vi "PMAC3000 SetUpDeviceOnUSB.vi"(0 "RD/WR Timeouts":i32=100, 1 "Software Number":string, 2 "VersionNumbers":string[](array[string]), 5 "Latency Timer":u8=8, 7 "Data Set-Up":T1={"Baud Rate"=1250000, "DataBits"=0, "StopBits"=0, "Parity"=0} {"Parity" items=["PARITY_NONE", "PARITY_ODD", "PARITY_EVEN", "PARITY_MARK", "PARITY_SPACE"]; "StopBits" items=["STOP_BITS_1", "STOP_BITS_1_5", "STOP_BITS_2"]; "DataBits" items=["BITS_5"=5, "BITS_6"=6, "BITS_7"=7, "BITS_8"=8]}, 9 "Flow Control Input":cluster{"FlowControl":u16, "Xon":u8, "Xoff":u8} {"FlowControl" items=["FLOW_NONE"=0, "FLOW_RTS_CTS"=256, "FLOW_DTR_DSR"=512, "FLOW_XON_OFF"=1024]}, 11 "Show Not Found Message":bool=TRUE, 12 "error in (no error)":errorcluster) -> (4 "USB Device Found":bool, 6 "USB Handle":i32, 8 "error out":errorcluster, 10 "NumberOfUsbDevices":i32, 14 "SoftwareVersionFound":string, 15 "Error":i32)   [LabVIEW 2018]
uses:
  ftd2xx.dll
panel:
  in  "FlowControl":u16(ring) items=["FLOW_NONE"=0, "FLOW_RTS_CTS"=256, "FLOW_DTR_DSR"=512, "FLOW_XON_OFF"=1024]
  in  "Parity":u8(ring) items=["PARITY_NONE", "PARITY_ODD", "PARITY_EVEN", "PARITY_MARK", "PARITY_SPACE"]
  in  "StopBits":u8(ring) items=["STOP_BITS_1", "STOP_BITS_1_5", "STOP_BITS_2"]
  in  "DataBits":u8(ring) items=["BITS_5"=5, "BITS_6"=6, "BITS_7"=7, "BITS_8"=8]
  out "Flags":i32
  out "Show Message":bool
  in  "Xoff":u8
  in  "Xon":u8
  in  "Baud Rate":i32=1250000
  out "Device Index":i32
  out "Number of Devices":i32
  # "Inputs"
  # "Misc"
  # "Outputs"
  # "e"
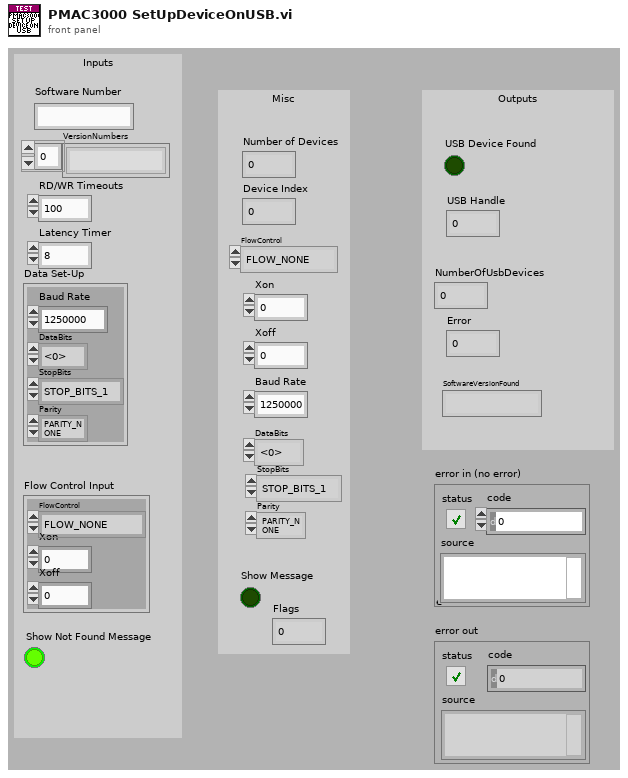
[diagram p1: front panel]
types:
  T1 = cluster{"Baud Rate":i32, "DataBits":u8, "StopBits":u8, "Parity":u8}
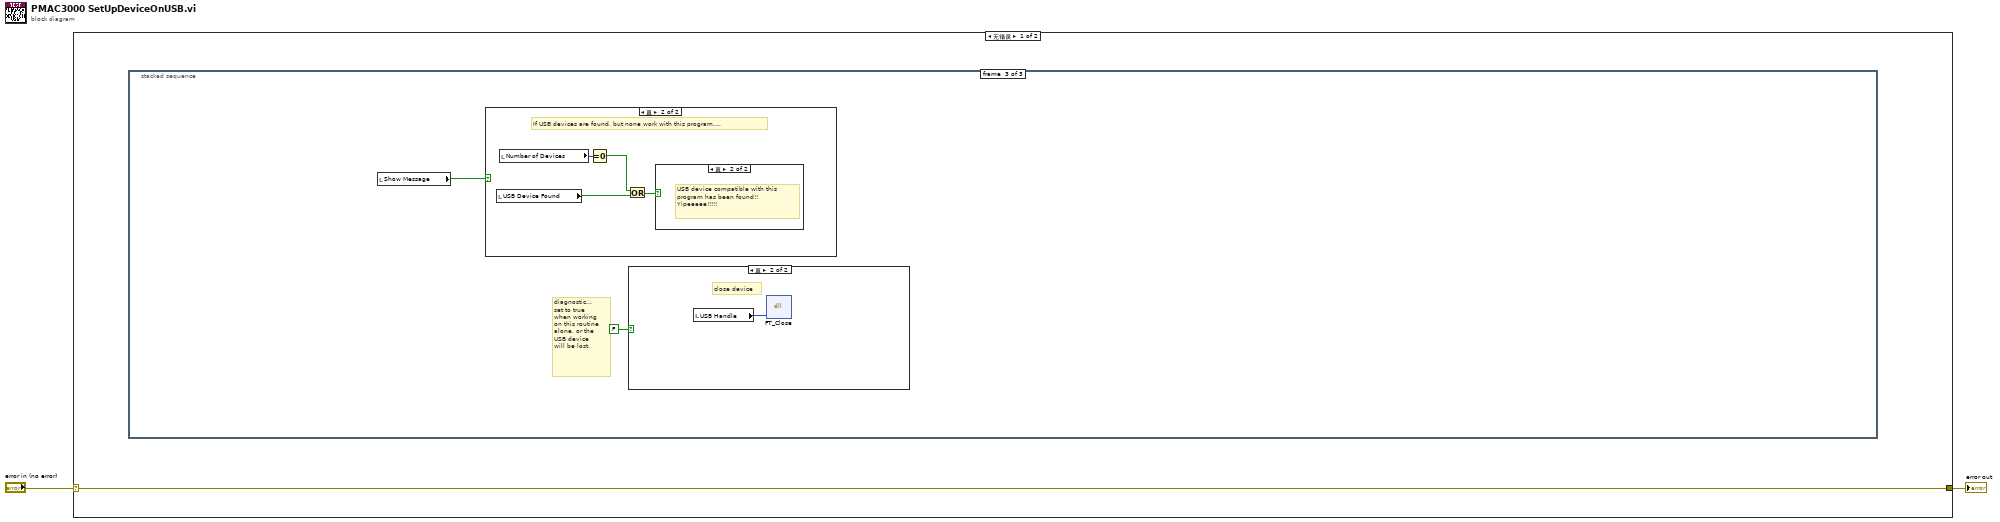
[diagram p0: block diagram]
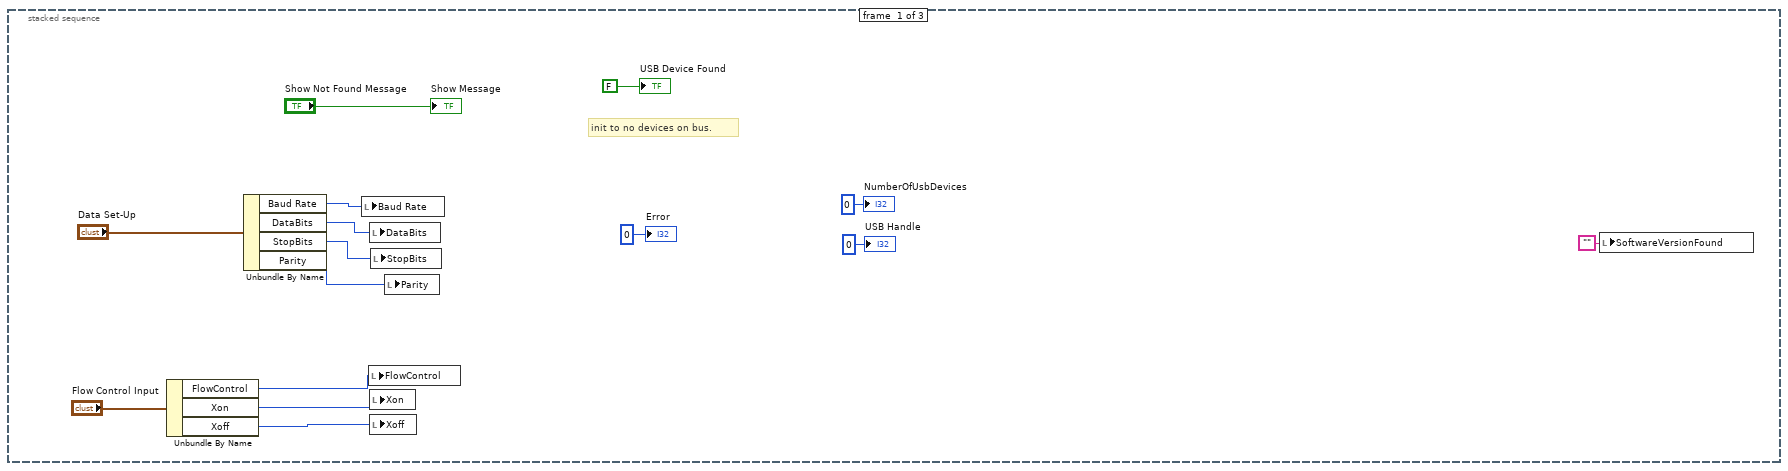
[diagram p2: hidden frame]
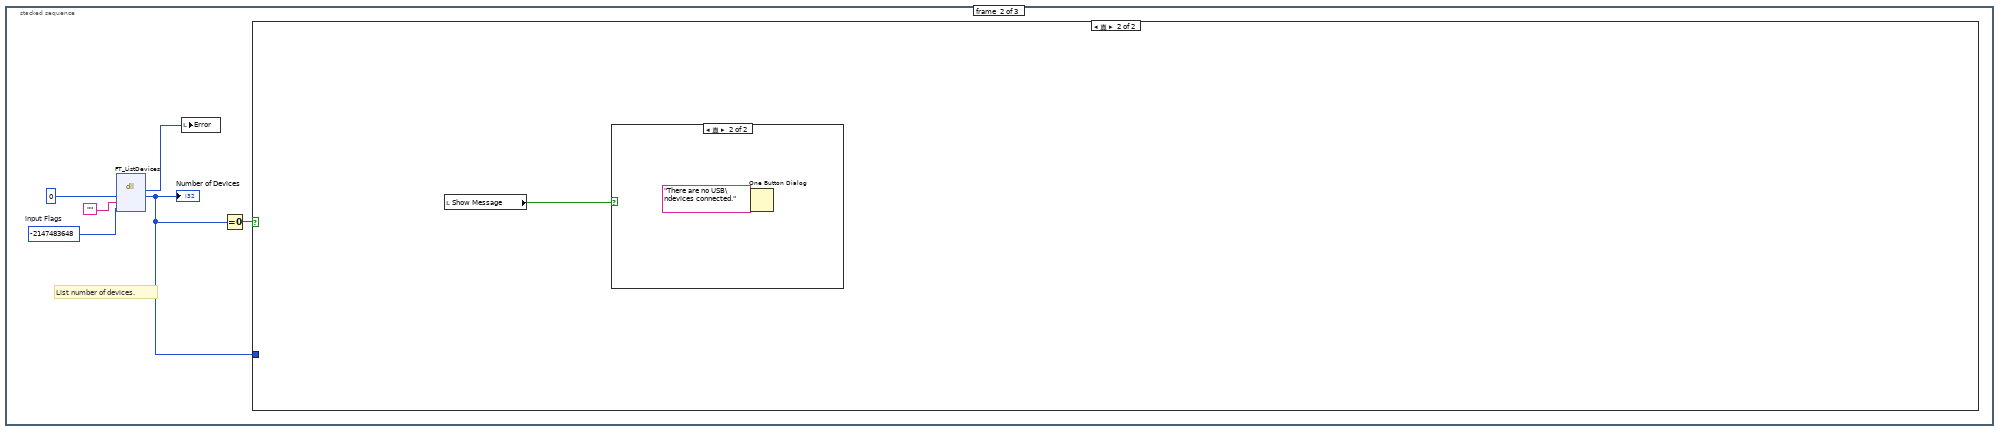
[diagram p3: hidden frame]
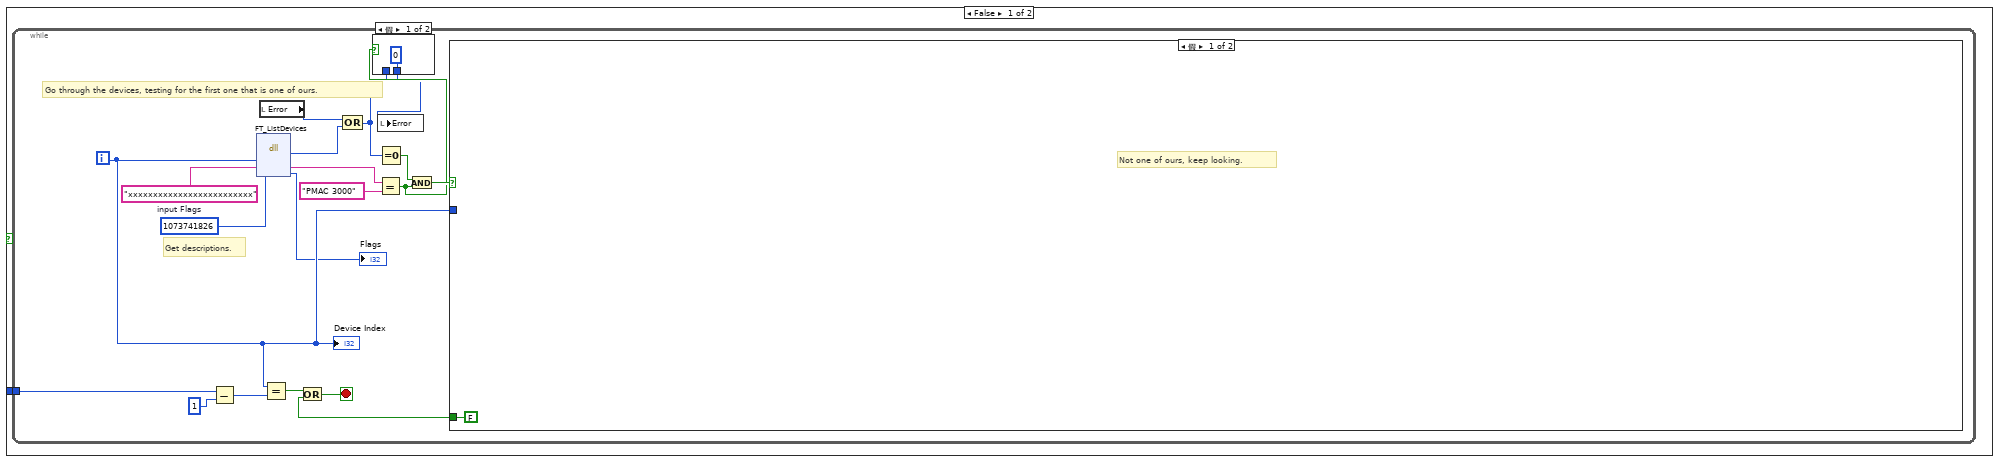
[diagram p4: hidden frame]
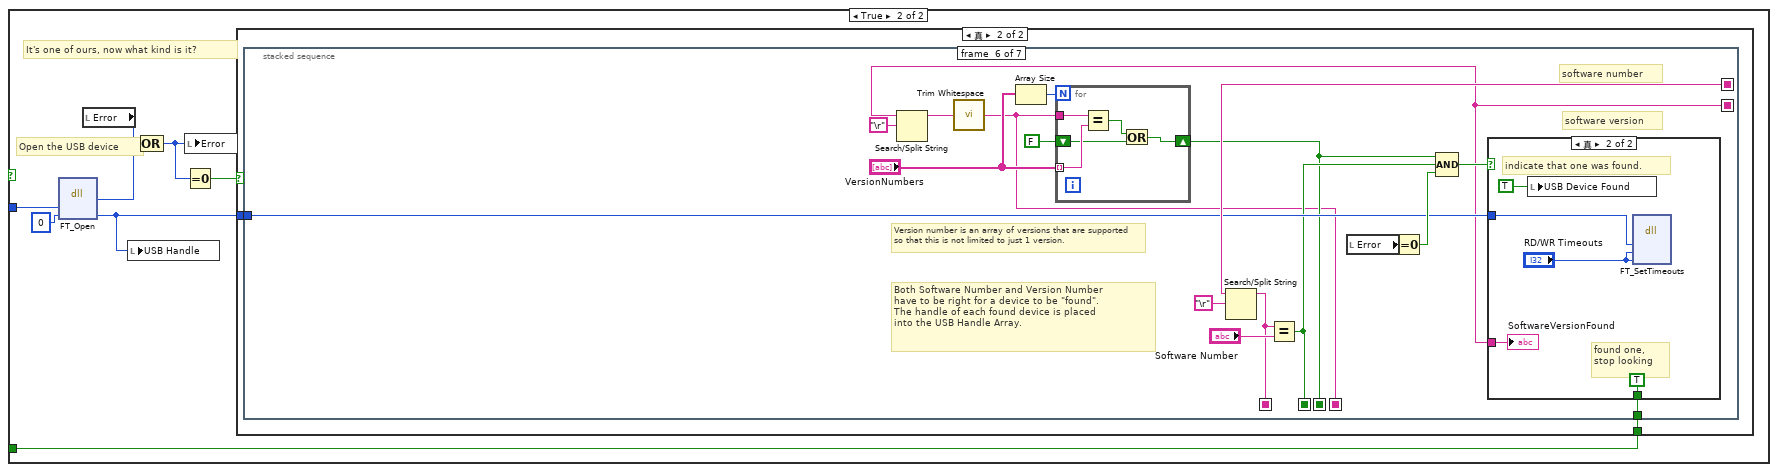
[diagram p6: hidden frame]
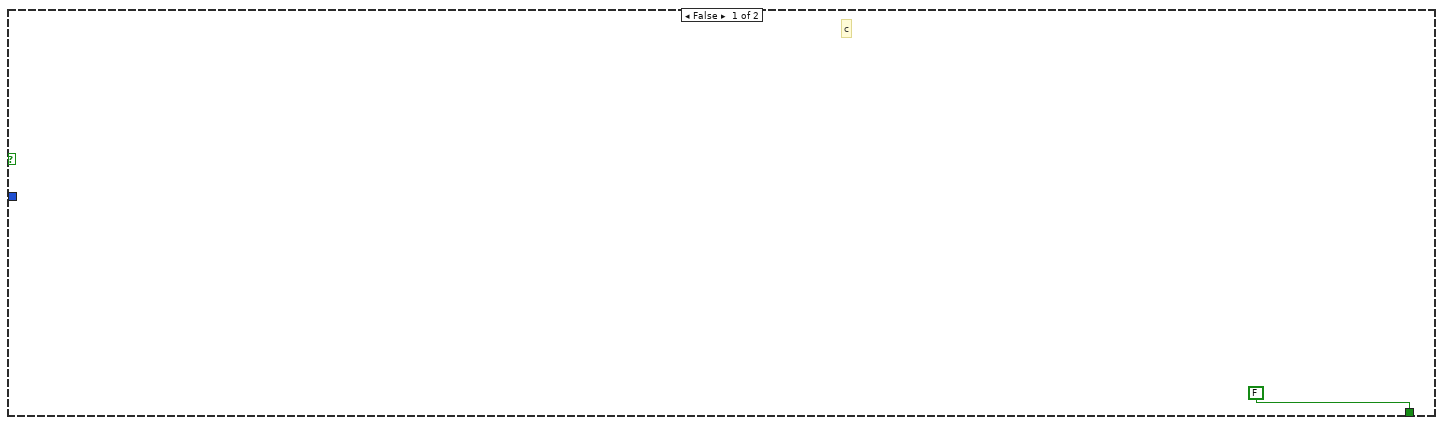
[diagram p7: hidden frame]
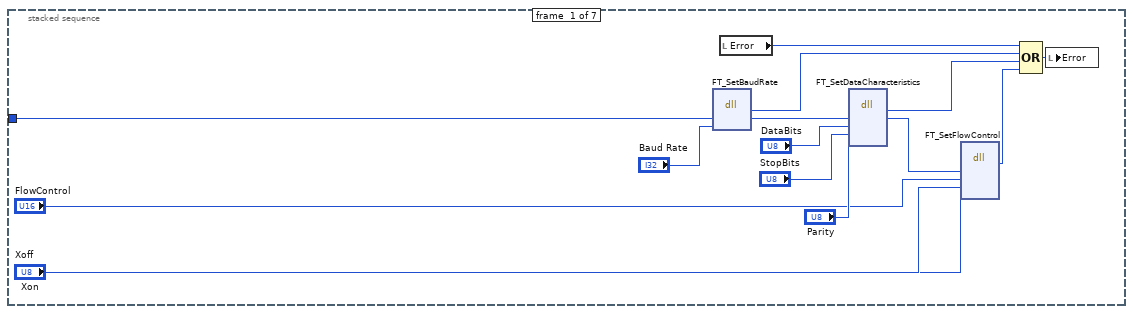
[diagram p8: hidden frame]
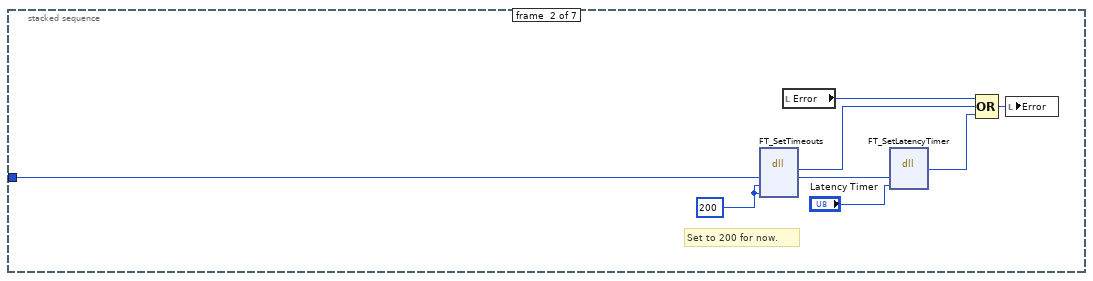
[diagram p9: hidden frame]
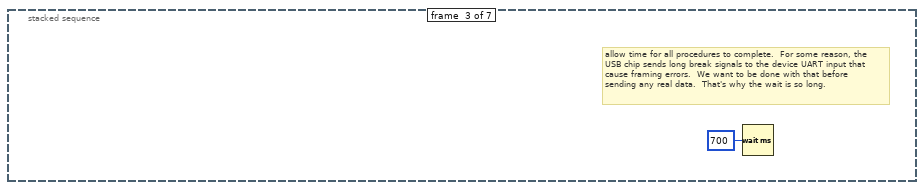
[diagram p10: hidden frame]
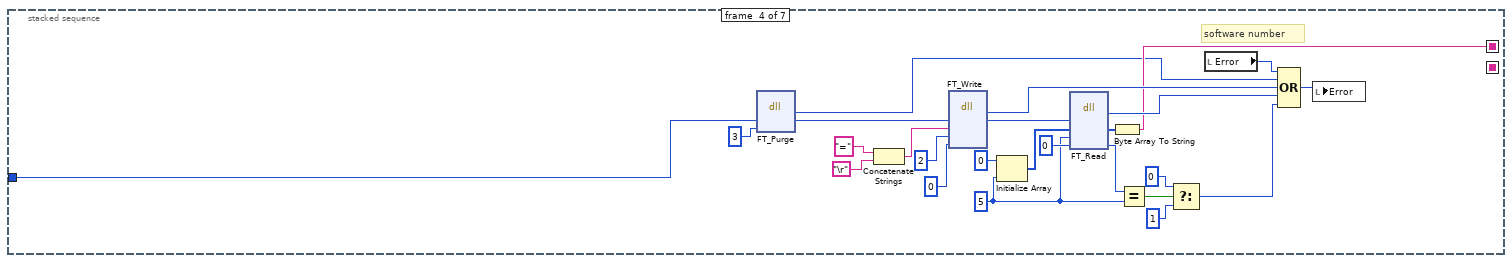
[diagram p11: hidden frame]
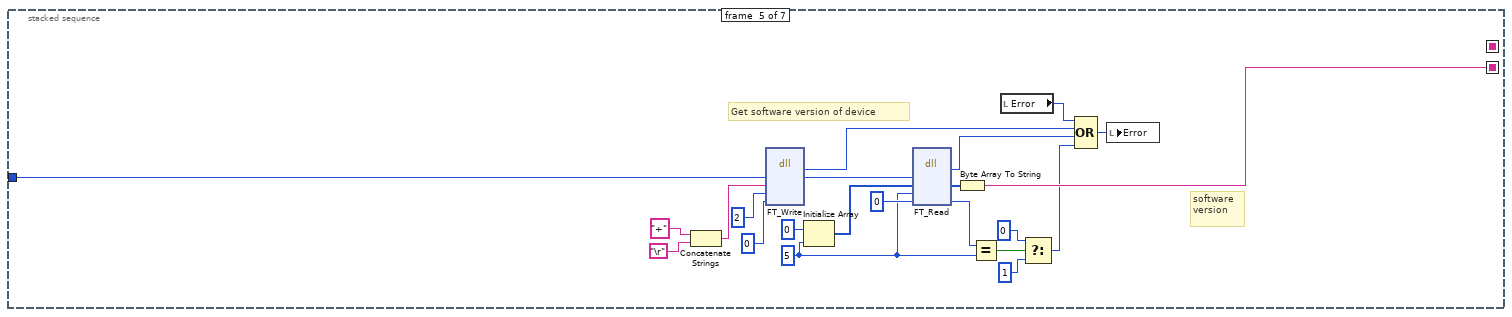
[diagram p12: hidden frame]
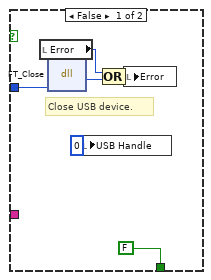
[diagram p13: hidden frame]
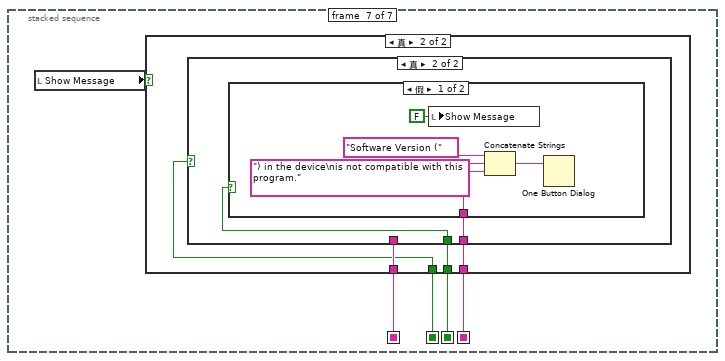
[diagram p14: hidden frame]
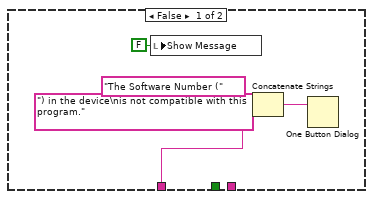
[diagram p16: hidden frame]
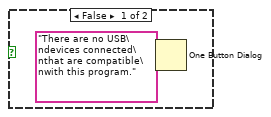
[diagram p20: hidden frame]
diagram:
  n1 = case shown="无错误" "error in (no error)" {
    selector: "error in (no error)" -> [w3 w195]
    tunnel: [w3 w195] -> w1
    frame No Error {
      n2 = stacked-sequence {
        frame #0 {
          # "init to no devices on bus."
          n3 = Unbundle By Name("Flow Control Input") -> ("FlowControl"=w6:u16, "Xon"=w5:u8, "Xoff"=w4:u8)
          n4 = Unbundle By Name("Data Set-Up") -> ("Baud Rate"=w11:i32, "DataBits"=w10:u8, "StopBits"=w9:u8, "Parity"=w8:u8)
          n5 = local write "Baud Rate"(w11) -> ()
          n6 = local write "FlowControl"(w6) -> ()
          n7 = local write "DataBits"(w10) -> ()
          n8 = local write "Xon"(w5) -> ()
          n9 = local write "Xoff"(w4) -> ()
          n10 = local write "StopBits"(w9) -> ()
          n11 = local write "Parity"(w8) -> ()
          n12 = local write "SoftwareVersionFound"("") -> ()
          "USB Device Found" <- FALSE ("USB Sensor Link Found")
          "Error" <- 0 ("Error")
          "Show Message" <- "Show Not Found Message"
          "NumberOfUsbDevices" <- 0 ("NumberOfUsbDevices")
          "USB Handle" <- 0 ("USB Handel")
        }
        frame #1 {
          w24 = -2147483648  # input Flags
          # "List number of devices."
          n13 = dll-call lib="C:/Labview Code/04.SubVI's/Others VI's/FTD2XX.dll" fn="FT_ListDevices"(0 ("input param"), "", "Flags"=w24) -> ("return type"=w19:i32, w21:i32)  [unwired: 5 in, 2 out]
          "Number of Devices" <- w21
          n14 = local write "Error"(w19) -> ()
          n15 = Equal To 0?(x=w21) -> (x = 0?=w23:bool)
          n16 = case shown="真" w23 {
            tunnel: w21 -> [w25 _]
            frame False {
              n17 = while {
                tunnel: w25 -> [w40]
                i -> [w38]
                stop <- w32 stop-if-true
                w43 = 1073741826  # input Flags
                # "Go through the devices, testing for the first one that is one of ours."
                # "Get descriptions."
                n18 = Subtract(x=w40, y=1) -> (x-y=w41:i32)
                n19 = dll-call lib="C:/Labview Code/04.SubVI's/Others VI's/FTD2XX.dll" fn="FT_ListDevices"(w38, "xxxxxxxxxxxxxxxxxxxxxxxxx" ("input param"), "Flags"=w43) -> ("return type"=w37:i32, w39:string, "Flags"=→"Flags":i32)  [unwired: 4 in, 2 out]
                n20 = local read "Error"() -> (w36:i32)
                n21 = Equal?(x=w38, y=w41) -> (x = y?=w33:bool)
                n22 = Compound Arithmetic op=OR(w36, w37) -> (w26:i32)
                n23 = Equal?(x=w39, y="PMAC 3000") -> (x = y?=w28:bool)
                n24 = case shown="假" w28 {
                  tunnel: [0 w46] -> w27
                  tunnel: w26 -> [_ w46]
                  frame False {
                  }
                  frame True {
                  }
                }
                n25 = local write "Error"(w27) -> ()
                n26 = Equal To 0?(x=w26) -> (x = 0?=w35:bool)
                n27 = And(x=w35, y=w28) -> (x .and. y?=w34:bool)
                n28 = case shown="假" w34 {
                  tunnel: w38 -> [_ w55]
                  tunnel: [FALSE w48] -> w31
                  frame False {
                    # "Not one of ours, keep looking."
                  }
                  frame True {
                    # "Open the USB device"
                    # "It's one of ours, now what kind is it?"
                    n29 = dll-call lib="C:/Labview Code/04.SubVI's/Others VI's/FTD2XX.dll" fn="FT_Open"(w55, "Handle"=0 ("input Handle")) -> ("return type"=w52:i32, "Handle"=w49:i32)  [unwired: 4 in, 2 out]
                    n30 = local read "Error"() -> (w53:i32)
                    n31 = local write "USB Handle"(w49) -> ()
                    n32 = Compound Arithmetic op=OR(w53, w52) -> (w50:i32)
                    n33 = local write "Error"(w50) -> ()
                    n34 = Equal To 0?(x=w50) -> (x = 0?=w51:bool)
                    n35 = case shown="真" w51 {
                      tunnel: w49 -> [_ w58]
                      tunnel: [FALSE w57] -> w48
                      frame False {
                        # "c"
                      }
                      frame True {
                        n36 = stacked-sequence {
                          seq-local: [_ _ _ w94 _ _ _] -> [_ _ _ _ _ w145 _]
                          seq-local: [_ _ _ _ w114 _ _] -> [_ _ _ _ _ w135 _]
                          seq-local: [_ _ _ _ _ w134 _] -> [_ _ _ _ _ _ w165]
                          seq-local: [_ _ _ _ _ w133 _] -> [_ _ _ _ _ _ w168]
                          seq-local: [_ _ _ _ _ w130 _] -> [_ _ _ _ _ _ w167]
                          seq-local: [_ _ _ _ _ w132 _] -> [_ _ _ _ _ _ w166]
                          tunnel: w58 -> [w63 w75 _ w93 w115 w140 _]
                          tunnel: [_ _ _ _ _ w139 _] -> w57
                          frame #0 {
                            n37 = dll-call lib="C:/Labview Code/04.SubVI's/Others VI's/FTD2XX.dll" fn="FT_SetBaudRate"("Handle"=w63, "BaudRate"="Baud Rate") -> ("return type"=w70:i32, "Handle"=w73:i32)  [unwired: 4 in, 2 out]
                            n38 = local read "Error"() -> (w69:i32)
                            n39 = dll-call lib="C:/Labview Code/04.SubVI's/Others VI's/FTD2XX.dll" fn="FT_SetDataCharacteristics"("Handle"=w73, "WordLength"="DataBits", "StopBits"="StopBits", "Parity"="Parity") -> ("return type"=w71:i32, "Handle"=w65:i32)  [unwired: 6 in, 2 out]
                            n40 = dll-call lib="C:/Labview Code/04.SubVI's/Others VI's/FTD2XX.dll" fn="FT_SetFlowControl"("Handle"=w65, "FlowControl"="FlowControl", "Xon"="Xon", "Xoff"="Xoff") -> ("return type"=w64:i32)  [unwired: 7 in, 2 out]
                            n41 = Compound Arithmetic op=OR(w69, w70, w71, w64) -> (w68:i32)
                            n42 = local write "Error"(w68) -> ()
                          }
                          frame #1 {
                            w74 = 200 ("RD/WR Timeouts")
                            # "Set to 200 for now."
                            n43 = dll-call lib="C:/Labview Code/04.SubVI's/Others VI's/FTD2XX.dll" fn="FT_SetTimeouts"("Handle"=w75, "ReadTimeout"=w74, "WriteTimeout"=w74) -> ("return type"=w78:i32, "Handle"=w81:i32)  [unwired: 5 in, 2 out]
                            n44 = local read "Error"() -> (w77:i32)
                            n45 = dll-call lib="C:/Labview Code/04.SubVI's/Others VI's/FTD2XX.dll" fn="FT_SetLatencyTimer"("Handle"=w81, "Timer"="Latency Timer") -> ("return type"=w79:i32)  [unwired: 5 in, 2 out]
                            n46 = Compound Arithmetic op=OR(w77, w78, w79) -> (w76:i32)
                            n47 = local write "Error"(w76) -> ()
                          }
                          frame #2 {
                            # "allow time for all procedures to complete.  For some reason, the\nUSB chip sends long break signals to the device UART input that\ncause framing errors.  We want to be done with that before\nsending any real data.  That's why the wait is so long."
                            n48 = Wait (ms)(milliseconds to wait=u32 700) -> ()  [unwired: 1 out]
                          }
                          frame #3 {
                            w87 = 5 ("dimension size")
                            # "software number"
                            n49 = dll-call lib="C:/Labview Code/04.SubVI's/Others VI's/FTD2XX.dll" fn="FT_Purge"("Handle"=w93, "Mask"=3) -> ("return type"=w90:i32, "Handle"=w92:i32)  [unwired: 4 in, 2 out]
                            n50 = Concatenate Strings("=" ("string"), "\r") -> (w106:string)
                            n51 = dll-call lib="C:/Labview Code/04.SubVI's/Others VI's/FTD2XX.dll" fn="FT_Write"("Handle"=w92, "Buffer"=w106, "BytesToWrite"=2, "BytesWritten"=0) -> ("return type"=w97:i32, "Handle"=w102:i32)  [unwired: 6 in, 2 out]
                            n52 = Initialize Array(u8 0 ("element"), w87) -> (w100:u8[])
                            n53 = dll-call lib="C:/Labview Code/04.SubVI's/Others VI's/FTD2XX.dll" fn="FT_Read"("Handle"=w102, "Buffer"=w100, "BytesToRead"=w87, "BytesReturned"=0) -> ("return type"=w96:i32, "Buffer"=w99:u8[], "BytesReturned"=w88:i32)  [unwired: 5 in, 2 out]
                            n54 = Byte Array To String(unsigned byte array=w99) -> (string=w94:string)
                            n55 = Equal?(x=w88, y=w87) -> (x = y?=w86:bool)
                            n56 = Select(t=0 ("BytesReturned"), s=w86, f=1) -> (s? t:f=w83:i32)
                            n57 = local read "Error"() -> (w89:i32)
                            n58 = Compound Arithmetic op=OR(w89, w90, w97, w96, w83) -> (w95:i32)
                            n59 = local write "Error"(w95) -> ()
                          }
                          frame #4 {
                            w110 = 5 ("dimension size")
                            # "software\nversion"
                            # "Get software version of device"
                            n60 = Concatenate Strings("+" ("string"), "\r") -> (w125:string)
                            n61 = dll-call lib="C:/Labview Code/04.SubVI's/Others VI's/FTD2XX.dll" fn="FT_Write"("Handle"=w115, "Buffer"=w125, "BytesToWrite"=2, "BytesWritten"=0) -> ("return type"=w119:i32, "Handle"=w121:i32)  [unwired: 6 in, 2 out]
                            n62 = Initialize Array(u8 0 ("element"), w110) -> (w123:u8[])
                            n63 = dll-call lib="C:/Labview Code/04.SubVI's/Others VI's/FTD2XX.dll" fn="FT_Read"("Handle"=w121, "Buffer"=w123, "BytesToRead"=w110, "BytesReturned"=0) -> ("return type"=w118:i32, "Buffer"=w129:u8[], "BytesReturned"=w109:i32)  [unwired: 5 in, 2 out]
                            n64 = Byte Array To String(unsigned byte array=w129) -> (string=w114:string)
                            n65 = Equal?(x=w109, y=w110) -> (x = y?=w113:bool)
                            n66 = local read "Error"() -> (w117:i32)
                            n67 = Select(t=0 ("BytesReturned"), s=w113, f=1) -> (s? t:f=w108:i32)
                            n68 = Compound Arithmetic op=OR(w117, w119, w118, w108) -> (w116:i32)
                            n69 = local write "Error"(w116) -> ()
                          }
                          frame #5 {
                            # "Version number is an array of versions that are supported\nso that this is not limited to just 1 version."
                            # "Both Software Number and Version Number\nhave to be right for a device to be \"found\".\nThe handle of each found device is placed\ninto the USB Handle Array."
                            # "software version"
                            # "software number"
                            n70 = Search/Split String(string=w135, search string/char (-)="\r") -> (substring before match=w131:string)  [unwired: 1 in, 2 out]
                            n71 = call <vilib>:"Trim Whitespace.vi"("string"=w131) -> ("trimmed string"=w130:string)  [unwired: 1 in]
                            n72 = Array Size(array="VersionNumbers") -> (size(s)=w137:i32)
                            n73 = for {
                              N: w137 -> [_]
                              tunnel: w130 -> [w152]
                              tunnel: "VersionNumbers" -> [w151] mode=indexing
                              shift-right: [w148] -> w133
                              shift-left: FALSE -> [w150]
                              n74 = Equal?(x=w152, y=w151) -> (x = y?=w149:bool)
                              n75 = Or(x=w149, y=w150) -> (x .or. y?=w148:bool)
                            }
                            n76 = Search/Split String(string=w145, search string/char (-)="\r") -> (substring before match=w132:string)  [unwired: 1 in, 2 out]
                            n77 = Equal?(x=w132, y="Software Number") -> (x = y?=w134:bool)
                            n78 = local read "Error"() -> (w142:i32)
                            n79 = Equal To 0?(x=w142) -> (x = 0?=w141:bool)
                            n80 = Compound Arithmetic op=AND(w133, w134, w141) -> (w143:bool)
                            n81 = case shown="真" w143 {
                              tunnel: w140 -> [w158 w159]
                              tunnel: [FALSE TRUE] -> w139
                              tunnel: w135 -> [_ w161]
                              frame False {
                                # "Close USB device."
                                n82 = local read "Error"() -> (w156:i32)
                                n83 = dll-call lib="C:/Labview Code/04.SubVI's/Others VI's/FTD2XX.dll" fn="FT_Close"("Handle"=w158) -> ("return type"=w157:i32)  [unwired: 4 in, 2 out]
                                n84 = local write "USB Handle"(0 ("USB Handle")) -> ()
                                n85 = Compound Arithmetic op=OR(w156, w157) -> (w155:i32)
                                n86 = local write "Error"(w155) -> ()
                              }
                              frame True {
                                # "found one,\nstop looking"
                                # "indicate that one was found."
                                n87 = local write "USB Device Found"(TRUE ("USB Sensor Link Found")) -> ()
                                n88 = dll-call lib="C:/Labview Code/04.SubVI's/Others VI's/FTD2XX.dll" fn="FT_SetTimeouts"("Handle"=w159, "ReadTimeout"="RD/WR Timeouts", "WriteTimeout"="RD/WR Timeouts") -> ()  [unwired: 7 in, 2 out]
                                "SoftwareVersionFound" <- w161
                              }
                            }
                          }
                          frame #6 {
                            n89 = local read "Show Message"() -> (w164:bool)
                            n90 = case shown="真" w164 {
                              tunnel: w168 -> [_ w172]
                              tunnel: w167 -> [_ w171]
                              tunnel: w166 -> [_ w170]
                              tunnel: w165 -> [_ w169]
                              frame False {
                              }
                              frame True {
                                n91 = case shown="真" w169 {
                                tunnel: w172 -> [_ w179]
                                tunnel: w171 -> [_ w178]
                                tunnel: w170 -> [w175 _]
                                frame False {
                                n92 = local write "Show Message"(FALSE ("Show Message")) -> ()
                                n93 = Concatenate Strings("The Software Number (" ("message"), w175, ") in the device\nis not compatible with this program." ("message")) -> (w173:string)
                                n94 = One Button Dialog(message=w173) -> ()  [unwired: 1 in, 1 out]
                                }
                                frame True {
                                n95 = case shown="假" w179 {
                                tunnel: w178 -> [w183 _]
                                frame False {
                                n96 = local write "Show Message"(FALSE ("Show Message")) -> ()
                                n97 = Concatenate Strings("Software Version (" ("string"), w183, ") in the device\nis not compatible with this program." ("string")) -> (w181:string)
                                n98 = One Button Dialog(message=w181) -> ()  [unwired: 1 in, 1 out]
                                }
                                frame True {
                                }
                                }
                                }
                                }
                              }
                            }
                          }
                        }
                      }
                    }
                  }
                }
                n99 = Or(x=w33, y=w31) -> (x .or. y?=w32:bool)
                "Device Index" <- w38
              }
            }
            frame True {
              n100 = local read "Show Message"() -> (w185:bool)
              n101 = case shown="真" w185 {
                frame False {
                }
                frame True {
                  n102 = One Button Dialog(message="There are no USB\ndevices connected.") -> ()  [unwired: 1 in, 1 out]
                }
              }
            }
          }
        }
        frame #2 {
          # "diagnostic...\nset to true\nwhen working\non this routine\nalone, or the\nUSB device\nwill be lost."
          n103 = local read "Show Message"() -> (w188:bool)
          n104 = case shown="真" w188 {
            frame False {
            }
            frame True {
              # "If USB devices are found, but none work with this program...."
              n105 = local read "USB Device Found"() -> (w189:bool)
              n106 = local read "Number of Devices"() -> (w192:i32)
              n107 = Equal To 0?(x=w192) -> (x = 0?=w190:bool)
              n108 = Or(x=w190, y=w189) -> (x .or. y?=w191:bool)
              n109 = case shown="真" w191 {
                frame False {
                  n110 = One Button Dialog(message="There are no USB\ndevices connected\nthat are compatible\nwith this program.") -> ()  [unwired: 1 in, 1 out]
                }
                frame True {
                  # "USB device compatible with this\nprogram has been found!!\nYipeeeee!!!!!"
                }
              }
            }
          }
          n111 = case shown="真" FALSE {
            frame False {
            }
            frame True {
              # "close device"
              n112 = local read "USB Handle"() -> (w194:i32)
              n113 = dll-call lib="C:/Labview Code/04.SubVI's/Others VI's/FTD2XX.dll" fn="FT_Close"("Handle"=w194) -> ()  [unwired: 5 in, 2 out]
            }
          }
        }
      }
    }
    frame Error {
    }
  }
  "error out" <- w1
